vi "Phasor Explorer Update UC Lifetimes.vi"(8 "Error In":errorcluster, 9 "Harmonic Frequency":dbl[unit], 10 "PhXP UC Plot Info in":T1={"Lifetime/Fraction Array"=[], "Phasor Explorer Parameters"={"Display Parameters"={"# Points"=0, "Ramp Type"=enum."Linear", "Type of Series"=enum."1-Exp Decays", "Min tau"=0.0, "Max tau"=0.0, "Include 0"=FALSE, "Include Infinity"=FALSE}, "Phasor Parameters"={"Harmonic Frequency"=0.0, "Use f* = 1/D Frequency"=FALSE, "Calibrated Phasor"=FALSE, "Calibration Lifetime"=1e-09, "Phasor Calculation"=enum."Direct Sum", "SEPL Type"=enum."UC", "# Gates"=1.0, "Square Gate Width"=1e-09, "Show Ticks"=FALSE}, "Decay & IRF Parameters"={"Lifetime"=0.0, "IRF Offset"=0.0, "IRF Period"=0.0, "Normalized Decays"=FALSE, "IRF Model"=enum."Dirac", "IRF Parameter 1"=0.0}, "Gate Parameters"={"First Gate Start"=0.0, "Use Gate Center"=FALSE, "Gate Width"=0.0, "Gate Step"=0.0, "# Gates"=0.0, "Gate Type"=enum."Square", "Edge Width"=0.0, "Top Slope"=0.0, "Reversed Sawtooth?"=FALSE, "Analytical Computation"=FALSE, "Integration"=enum."Item 0", "Tolerance"=1.0, "# Steps"=1.0, "Type of User-defined Function"=enum."Gate", "Use Gate Step"=FALSE}, "Detector Parameters"={"Frames/Image"=0, "Gates/Frame"=0, "Bits/Frame"=0, "Multiplicity"=0, "Incident Signal"=0.0, "Poisson Signal"=FALSE}}, "Phase Lifetimes"=[], "Modulus Lifetimes"=[]} {"Phasor Explorer Parameters"."Detector Parameters"."Frames/Image" min=1; "Phasor Explorer Parameters"."Detector Parameters"."Multiplicity" min=0; "Phasor Explorer Parameters"."Detector Parameters"."Bits/Frame" min=1; "Phasor Explorer Parameters"."Detector Parameters"."Gates/Frame" min=1; "Phasor Explorer Parameters"."Gate Parameters"."# Steps" min=0.0; "Phasor Explorer Parameters"."Gate Parameters"."Tolerance" min=0.0; "Phasor Explorer Parameters"."Gate Parameters"."Top Slope" min=0.0; "Phasor Explorer Parameters"."Gate Parameters"."Edge Width" min=0.0; "Phasor Explorer Parameters"."Gate Parameters"."Gate Step" min=0.0; "Phasor Explorer Parameters"."Gate Parameters"."# Gates" min=0.0 step=1.0; "Phasor Explorer Parameters"."Gate Parameters"."Gate Width" min=0.0; "Phasor Explorer Parameters"."Decay & IRF Parameters"."Lifetime" min=0.0; "Phasor Explorer Parameters"."Decay & IRF Parameters"."IRF Period" min=0.0; "Phasor Explorer Parameters"."Phasor Parameters"."Square Gate Width" min=0.0; "Phasor Explorer Parameters"."Phasor Parameters"."# Gates" min=0.0; "Phasor Explorer Parameters"."Phasor Parameters"."Calibration Lifetime" min=0.0; "Phasor Explorer Parameters"."Phasor Parameters"."Harmonic Frequency" min=0.0; "Phasor Explorer Parameters"."Display Parameters"."Min tau" min=0.0; "Phasor Explorer Parameters"."Display Parameters"."Max tau" min=0.0; "Phasor Explorer Parameters"."Display Parameters"."# Points" min=1 step=1}, 11 "Universal Semi-circle":cluster{"X Array":dbl[], "Y Array":dbl[]}) -> (0 "Error Out":errorcluster, 2 "PhXP UC Plot Info out":T1={"Lifetime/Fraction Array"=[], "Phasor Explorer Parameters"={"Display Parameters"={"# Points"=0, "Ramp Type"=enum."Linear", "Type of Series"=enum."1-Exp Decays", "Min tau"=0.0, "Max tau"=0.0, "Include 0"=FALSE, "Include Infinity"=FALSE}, "Phasor Parameters"={"Harmonic Frequency"=0.0, "Use f* = 1/D Frequency"=FALSE, "Calibrated Phasor"=FALSE, "Calibration Lifetime"=1e-09, "Phasor Calculation"=enum."Direct Sum", "SEPL Type"=enum."UC", "# Gates"=1.0, "Square Gate Width"=1e-09, "Show Ticks"=FALSE}, "Decay & IRF Parameters"={"Lifetime"=0.0, "IRF Offset"=0.0, "IRF Period"=0.0, "Normalized Decays"=FALSE, "IRF Model"=enum."Dirac", "IRF Parameter 1"=0.0}, "Gate Parameters"={"First Gate Start"=0.0, "Use Gate Center"=FALSE, "Gate Width"=0.0, "Gate Step"=0.0, "# Gates"=0.0, "Gate Type"=enum."Square", "Edge Width"=0.0, "Top Slope"=0.0, "Reversed Sawtooth?"=FALSE, "Analytical Computation"=FALSE, "Integration"=enum."Item 0", "Tolerance"=1.0, "# Steps"=1.0, "Type of User-defined Function"=enum."Gate", "Use Gate Step"=FALSE}, "Detector Parameters"={"Frames/Image"=0, "Gates/Frame"=0, "Bits/Frame"=0, "Multiplicity"=0, "Incident Signal"=0.0, "Poisson Signal"=FALSE}}, "Phase Lifetimes"=[], "Modulus Lifetimes"=[]} {"Phasor Explorer Parameters"."Detector Parameters"."Frames/Image" min=1; "Phasor Explorer Parameters"."Detector Parameters"."Multiplicity" min=0; "Phasor Explorer Parameters"."Detector Parameters"."Bits/Frame" min=1; "Phasor Explorer Parameters"."Detector Parameters"."Gates/Frame" min=1; "Phasor Explorer Parameters"."Gate Parameters"."# Steps" min=0.0; "Phasor Explorer Parameters"."Gate Parameters"."Tolerance" min=0.0; "Phasor Explorer Parameters"."Gate Parameters"."Top Slope" min=0.0; "Phasor Explorer Parameters"."Gate Parameters"."Edge Width" min=0.0; "Phasor Explorer Parameters"."Gate Parameters"."Gate Step" min=0.0; "Phasor Explorer Parameters"."Gate Parameters"."# Gates" min=0.0 step=1.0; "Phasor Explorer Parameters"."Gate Parameters"."Gate Width" min=0.0; "Phasor Explorer Parameters"."Decay & IRF Parameters"."Lifetime" min=0.0; "Phasor Explorer Parameters"."Decay & IRF Parameters"."IRF Period" min=0.0; "Phasor Explorer Parameters"."Phasor Parameters"."Square Gate Width" min=0.0; "Phasor Explorer Parameters"."Phasor Parameters"."# Gates" min=0.0; "Phasor Explorer Parameters"."Phasor Parameters"."Calibration Lifetime" min=0.0; "Phasor Explorer Parameters"."Phasor Parameters"."Harmonic Frequency" min=0.0; "Phasor Explorer Parameters"."Display Parameters"."Min tau" min=0.0; "Phasor Explorer Parameters"."Display Parameters"."Max tau" min=0.0; "Phasor Explorer Parameters"."Display Parameters"."# Points" min=1 step=1})   [LabVIEW 2019]
uses:
  Phasor Explorer Phasor Plot Info.ctl
  SEPL Parameters.ctl
  Phasor Explorer Display Parameters.ctl
  Type of Series.ctl
  Phasor Explorer Phasor Parameters.ctl
  Phasor Calculation Type.ctl
  SEPL Type.ctl
  Phasor Explorer Decay Parameters.ctl
  IRF Model.ctl
  Phasor Explorer Gate Parameters.ctl
  Gate Type.ctl
  Type of User-defined Function.ctl
  Phasor Explorer Detector Parameters.ctl
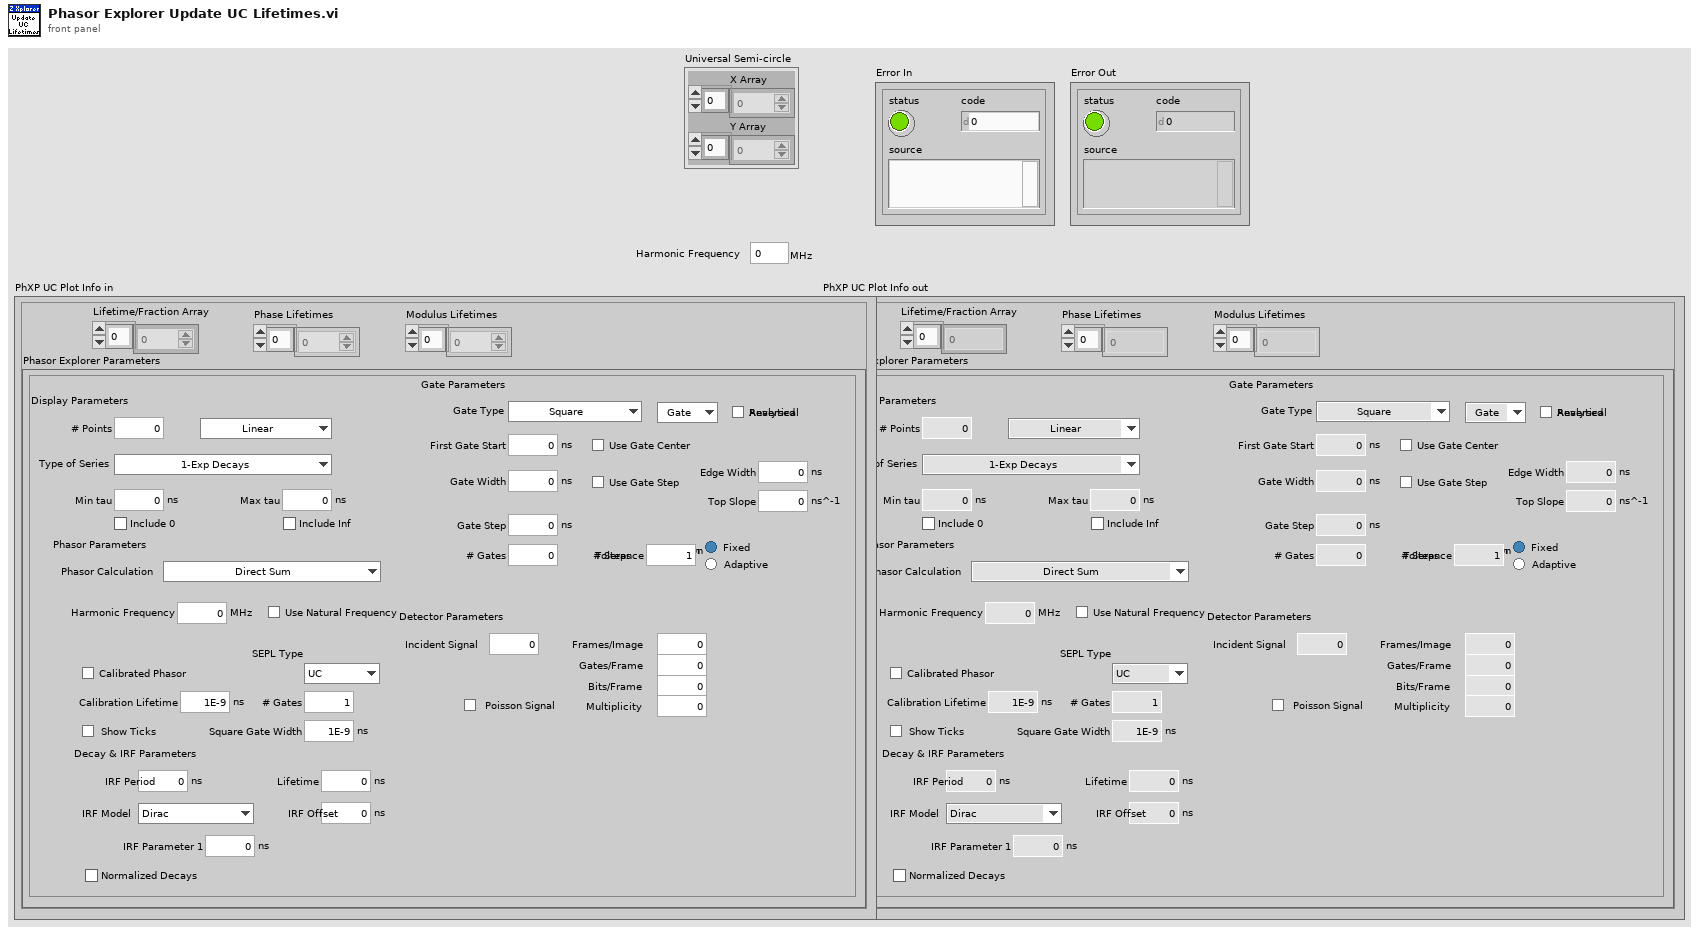
[diagram p1: front panel]
types:
  T1 = typedef "Phasor Explorer Phasor Plot Info.ctl" = cluster{"Lifetime/Fraction Array":dbl[], "Phasor Explorer Parameters":T2, "Phase Lifetimes":dbl[], "Modulus Lifetimes":dbl[]}
  T2 = typedef "SEPL Parameters.ctl" = cluster{"Display Parameters":T3, "Phasor Parameters":T5, "Decay & IRF Parameters":T8, "Gate Parameters":T10, "Detector Parameters":T13}
  T3 = typedef "Phasor Explorer Display Parameters.ctl" = cluster{"# Points":i32, "Ramp Type":enum16{"Linear", "Logarithmic"}, "Type of Series":T4, "Min tau":dbl[unit], "Max tau":dbl[unit], "Include 0":bool, "Include Infinity":bool}
  T4 = typedef "Type of Series.ctl" = enum16{"1-Exp Decays", "Linear Combination of 1-Exp"}
  T5 = typedef "Phasor Explorer Phasor Parameters.ctl" = cluster{"Harmonic Frequency":dbl[unit], "Use f* = 1/D Frequency":bool, "Calibrated Phasor":bool, "Calibration Lifetime":dbl[unit], "Phasor Calculation":T6, "SEPL Type":T7, "# Gates":dbl, "Square Gate Width":dbl[unit], "Show Ticks":bool}
  T6 = typedef "Phasor Calculation Type.ctl" = enum16{"Direct Sum", "Analytical Formula"}
  T7 = typedef "SEPL Type.ctl" = enum16{"UC", "L_N", "L_N[W]", "L_X"}
  T8 = typedef "Phasor Explorer Decay Parameters.ctl" = cluster{"Lifetime":dbl[unit], "IRF Offset":dbl[unit], "IRF Period":dbl[unit], "Normalized Decays":bool, "IRF Model":T9, "IRF Parameter 1":dbl[unit]}
  T9 = typedef "IRF Model.ctl" = enum16{"Dirac", "Exponential"}
  T10 = typedef "Phasor Explorer Gate Parameters.ctl" = cluster{"First Gate Start":dbl[unit], "Use Gate Center":bool, "Gate Width":dbl[unit], "Gate Step":dbl[unit], "# Gates":dbl, "Gate Type":T11, "Edge Width":dbl[unit], "Top Slope":dbl[unit], "Reversed Sawtooth?":bool, "Analytical Computation":bool, "Integration":enum32{"Item 0", "Item 1"}, "Tolerance":dbl, "# Steps":dbl, "Type of User-defined Function":T12, "Use Gate Step":bool}
  T11 = typedef "Gate Type.ctl" = enum16{"Square", "Finite Edge Square", "Finite Edge, Tilted Top Square", "Triangle", "Sawtooth", "User-defined"}
  T12 = typedef "Type of User-defined Function.ctl" = enum16{"Gate", "IRF"}
  T13 = typedef "Phasor Explorer Detector Parameters.ctl" = cluster{"Frames/Image":i32, "Gates/Frame":i32, "Bits/Frame":i32, "Multiplicity":i32, "Incident Signal":dbl, "Poisson Signal":bool}
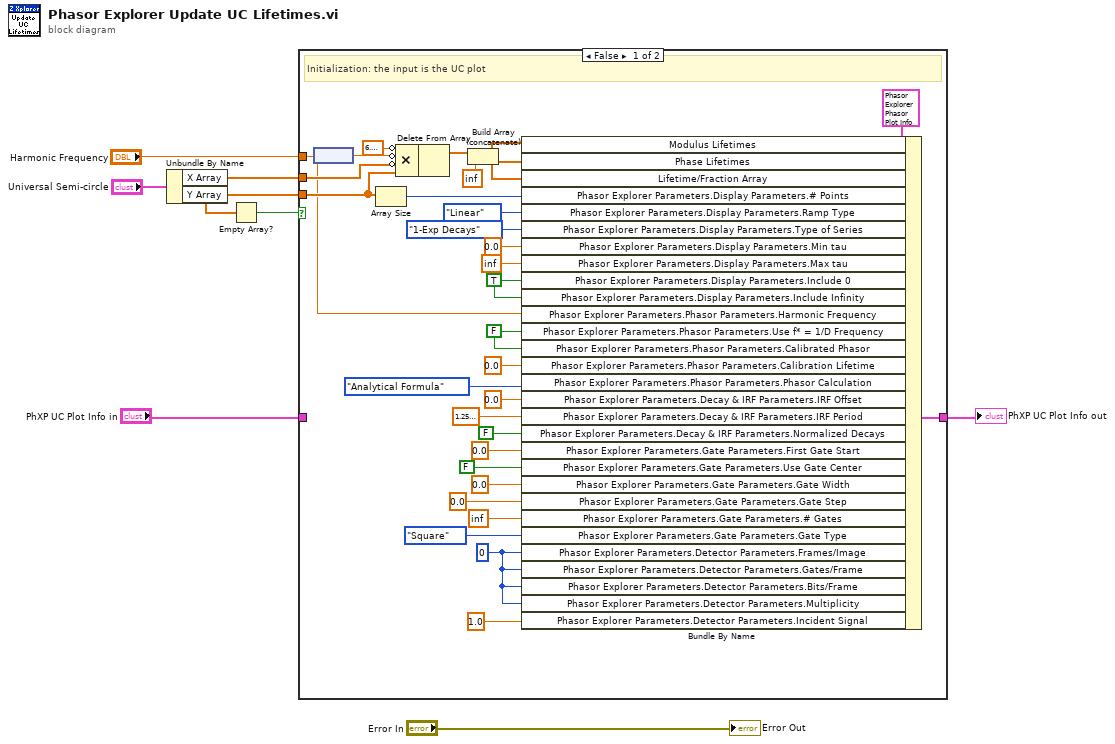
[diagram p0: block diagram]
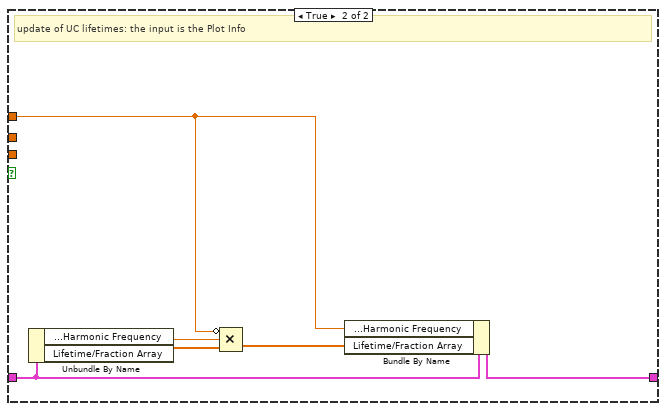
[diagram p2: hidden frame]
diagram:
  n1 = Unbundle By Name("Universal Semi-circle") -> ("X Array"=w7:dbl[], "Y Array"=w5:dbl[])
  n2 = Empty Array?(array=w5) -> (empty?=w4:bool)
  n3 = case shown="False" w4 {
    tunnel: w7 -> [w18 _]
    tunnel: "Harmonic Frequency" -> [w9 w40]
    tunnel: [w15 w41] -> w6
    tunnel: w5 -> [w14 _]
    tunnel: "PhXP UC Plot Info in" -> [_ w43]
    frame False {
      w25 = 0 ("Phasor Explorer Parameters.Detector Parameters.Frames/Image: F")
      w37 = FALSE ("Phasor Explorer Parameters.Phasor Parameters.Use Natural Frequency")
      w38 = TRUE ("Phasor Explorer Parameters.Display Parameters.Include 0")
      # "Initialization: the input is the UC plot"
      n4 = node(w9) -> (w13:dbl)
      n5 = Array Size(array=w14) -> (size(s)=w19:i32)
      n6 = Compound Arithmetic op=MULTIPLY(invert 6.283185307179586, invert w13, invert w18, w14) -> (w16:dbl[])
      n7 = Delete From Array(array=w16) -> (array with subset deleted=w12:dbl[])  [unwired: 2 in, 1 out]
      n8 = Build Array (concatenate)(w12, inf ("element")) -> (w10:dbl[])
      n9 = Bundle By Name(cluster=T1 {"Lifetime/Fraction Array"=[], "Phasor Explorer Parameters"={"Display Parameters"={"# Points"=0, "Ramp Type"=enum."Linear", "Type of Series"=enum."1-Exp Decays", "Min tau"=0.0, "Max tau"=0.0, "Include 0"=FALSE, "Include Infinity"=FALSE}, "Phasor Parameters"={"Harmonic Frequency"=0.0, "Use f* = 1/D Frequency"=FALSE, "Calibrated Phasor"=FALSE, "Calibration Lifetime"=0.0, "Phasor Calculation"=enum."Direct Sum", "SEPL Type"=enum."UC", "# Gates"=1.0, "Square Gate Width"=1e-09, "Show Ticks"=FALSE}, "Decay & IRF Parameters"={"Lifetime"=0.0, "IRF Offset"=0.0, "IRF Period"=0.0, "Normalized Decays"=FALSE, "IRF Model"=enum."Dirac", "IRF Parameter 1"=0.0}, "Gate Parameters"={"First Gate Start"=0.0, "Use Gate Center"=FALSE, "Gate Width"=0.0, "Gate Step"=0.0, "# Gates"=0.0, "Gate Type"=enum."Square", "Edge Width"=0.0, "Top Slope"=0.0, "Reversed Sawtooth?"=FALSE, "Analytical Computation"=FALSE, "Integration"=enum."Item 0", "Tolerance"=1.0, "# Steps"=1.0, "Type of User-defined Function"=enum."Gate", "Use Gate Step"=FALSE}, "Detector Parameters"={"Frames/Image"=0, "Gates/Frame"=0, "Bits/Frame"=0, "Multiplicity"=0, "Incident Signal"=0.0, "Poisson Signal"=FALSE}}, "Phase Lifetimes"=[], "Modulus Lifetimes"=[]} ("Phasor Graph Plot Info"), "Modulus Lifetimes"=w10, "Phase Lifetimes"=w10, "Lifetime/Fraction Array"=w10, "Phasor Explorer Parameters.Display Parameters.# Points"=w19, "Phasor Explorer Parameters.Display Parameters.Ramp Type"=enum16{"Linear", "Logarithmic"}."Linear", "Phasor Explorer Parameters.Display Parameters.Type of Series"=Type_of_Series."1-Exp Decays", "Phasor Explorer Parameters.Display Parameters.Min tau"=dbl[unit] 0.0, "Phasor Explorer Parameters.Display Parameters.Max tau"=dbl[unit] inf, "Phasor Explorer Parameters.Display Parameters.Include 0"=w38, "Phasor Explorer Parameters.Display Parameters.Include Infinity"=w38, "Phasor Explorer Parameters.Phasor Parameters.Harmonic Frequency"=w9, "Phasor Explorer Parameters.Phasor Parameters.Use f* = 1/D Frequency"=w37, "Phasor Explorer Parameters.Phasor Parameters.Calibrated Phasor"=w37, "Phasor Explorer Parameters.Phasor Parameters.Calibration Lifetime"=dbl[unit] 0.0, "Phasor Explorer Parameters.Phasor Parameters.Phasor Calculation"=Phasor_Calculation_Type."Analytical Formula", "Phasor Explorer Parameters.Decay & IRF Parameters.IRF Offset"=dbl[unit] 0.0 ("Phasor Explorer Parameters.Decay Parameters.Offset"), "Phasor Explorer Parameters.Decay & IRF Parameters.IRF Period"=dbl[unit] 1.2500000000000001e-08 ("Phasor Explorer Parameters.Decay Parameters.Period"), "Phasor Explorer Parameters.Decay & IRF Parameters.Normalized Decays"=FALSE ("Phasor Explorer Parameters.Decay Parameters.Normalized Decays"), "Phasor Explorer Parameters.Gate Parameters.First Gate Start"=dbl[unit] 0.0, "Phasor Explorer Parameters.Gate Parameters.Use Gate Center"=FALSE, "Phasor Explorer Parameters.Gate Parameters.Gate Width"=dbl[unit] 0.0, "Phasor Explorer Parameters.Gate Parameters.Gate Step"=dbl[unit] 0.0, "Phasor Explorer Parameters.Gate Parameters.# Gates"=inf, "Phasor Explorer Parameters.Gate Parameters.Gate Type"=Gate_Type."Square", "Phasor Explorer Parameters.Detector Parameters.Frames/Image"=w25, "Phasor Explorer Parameters.Detector Parameters.Gates/Frame"=w25, "Phasor Explorer Parameters.Detector Parameters.Bits/Frame"=w25, "Phasor Explorer Parameters.Detector Parameters.Multiplicity"=w25, "Phasor Explorer Parameters.Detector Parameters.Incident Signal"=1.0 ("Phasor Explorer Parameters.Detector Parameters.Incident Signal: I")) -> (w15:T1)
    }
    frame True {
      # "update of UC lifetimes: the input is the Plot Info"
      n10 = Unbundle By Name(w43) -> ("Phasor Explorer Parameters.Phasor Parameters.Harmonic Frequency"=w44:dbl[unit], "Lifetime/Fraction Array"=w45:dbl[])
      n11 = Compound Arithmetic op=MULTIPLY(invert w40, w44, w45) -> (w42:dbl[])
      n12 = Bundle By Name(cluster=w43, "Phasor Explorer Parameters.Phasor Parameters.Harmonic Frequency"=w40, "Lifetime/Fraction Array"=w42) -> (w41:T1)
    }
  }
  "PhXP UC Plot Info out" <- w6
  "Error Out" <- "Error In"
